vi "BBB_ParseString.vi"(8 "Input String":string) -> (1 "Spectral Data":dbl[](array[numeric]), 2 "Data out":T1, 3 "file name":string, 5 "BBB Timestamp":timestamp)   [LabVIEW 2025]
uses:
  TypeDef_DataIn.ctl
panel:
  in  "Data in":T1
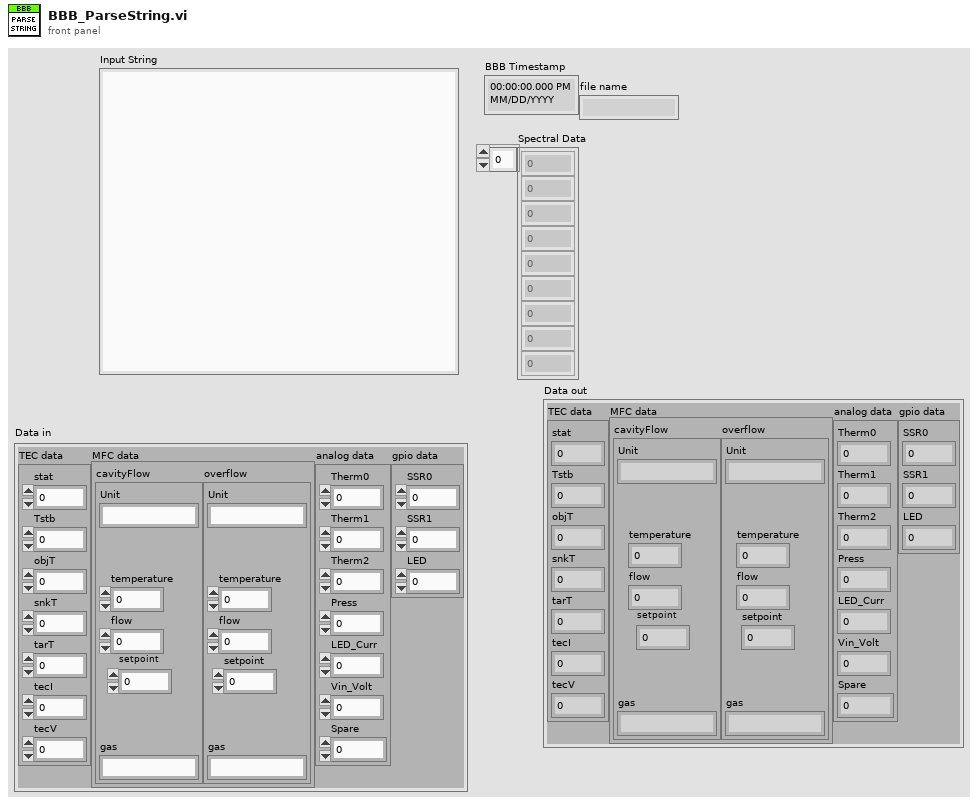
[diagram p1: front panel]
types:
  T1 = typedef "TypeDef_DataIn.ctl" = cluster{"TEC data":cluster{"stat":i32, "Tstb":i32, "objT":dbl, "snkT":dbl, "tarT":dbl, "tecI":dbl, "tecV":dbl}, "MFC data":cluster{"cavityFlow":cluster{"Unit":string, "temperature":dbl, "flow":dbl, "setpoint":dbl, "gas":string}, "overflow":cluster{"Unit":string, "temperature":dbl, "flow":dbl, "setpoint":dbl, "gas":string}}, "analog data":cluster{"Therm0":dbl, "Therm1":dbl, "Therm2":dbl, "Press":dbl, "LED_Curr":dbl, "Vin_Volt":dbl, "Spare":dbl}, "gpio data":cluster{"SSR0":i32, "SSR1":i32, "LED":i32}}
  T2 = cluster{"cavityFlow":cluster{"Unit":string, "temperature":dbl, "flow":dbl, "totalizer":dbl, "setpoint":dbl, "valve drive":dbl, "gas":string}, "overflow":cluster{"Unit":string, "temperature":dbl, "flow":dbl, "totalizer":dbl, "setpoint":dbl, "valve drive":dbl, "gas":string}}
  T3 = cluster{"stat":i32, "Tstb":i32, "objT":dbl, "snkT":dbl, "tarT":dbl, "tecI":dbl, "tecV":dbl}
  T4 = cluster{"cavityFlow":cluster{"Unit":string, "temperature":dbl, "flow":dbl, "setpoint":dbl, "gas":string}, "overflow":cluster{"Unit":string, "temperature":dbl, "flow":dbl, "setpoint":dbl, "gas":string}}
  T5 = cluster{"Therm0":dbl, "Therm1":dbl, "Therm2":dbl, "Press":dbl, "LED_Curr":dbl, "Vin_Volt":dbl, "Spare":dbl}
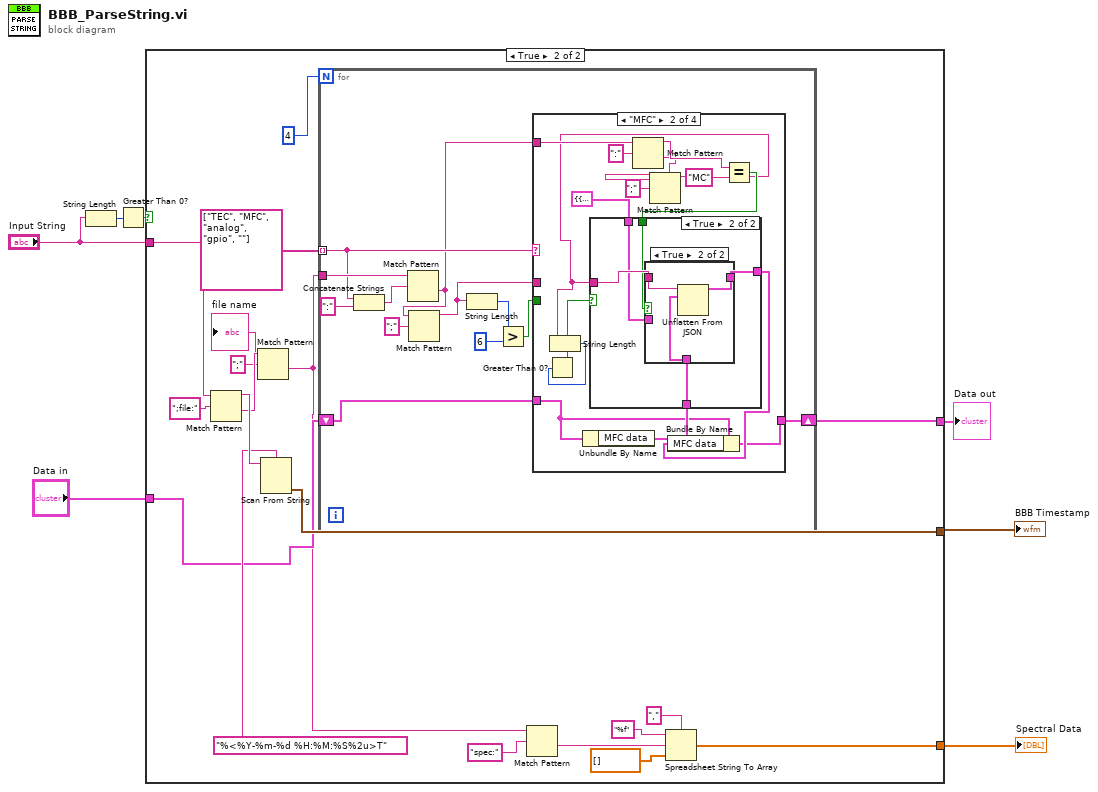
[diagram p0: block diagram]
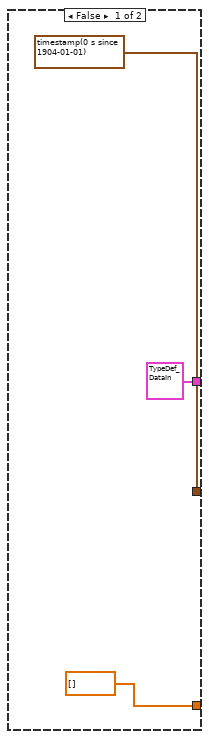
[diagram p2: hidden frame]
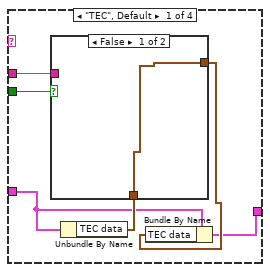
[diagram p3: hidden frame]
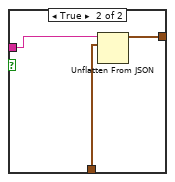
[diagram p4: hidden frame]
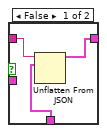
[diagram p6: hidden frame]
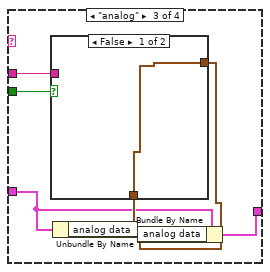
[diagram p7: hidden frame]
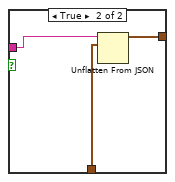
[diagram p8: hidden frame]
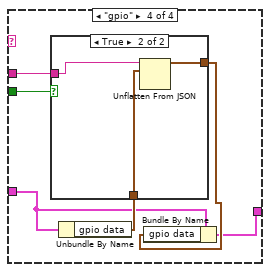
[diagram p9: hidden frame]
diagram:
  n1 = String Length(string="Input String") -> (length=w7:i32)
  n2 = Greater Than 0?(x=w7) -> (x > 0?=w6:bool)
  n3 = case shown="True" w6 {
    tunnel: "Input String" -> [_ w28]
    tunnel: [timestamp(0 s since 1904-01-01) w26] -> w4
    tunnel: [dbl[] [] ("array type (2D Dbl)") w17] -> w3
    tunnel: [T1 {"TEC data"={"stat"=0, "Tstb"=0, "objT"=0.0, "snkT"=0.0, "tarT"=0.0, "tecI"=0.0, "tecV"=0.0}, "MFC data"={"cavityFlow"={"Unit"="", "temperature"=0.0, "flow"=0.0, "setpoint"=0.0, "gas"=""}, "overflow"={"Unit"="", "temperature"=0.0, "flow"=0.0, "setpoint"=0.0, "gas"=""}}, "analog data"={"Therm0"=0.0, "Therm1"=0.0, "Therm2"=0.0, "Press"=0.0, "LED_Curr"=0.0, "Vin_Volt"=0.0, "Spare"=0.0}, "gpio data"={"SSR0"=0, "SSR1"=0, "LED"=0}} ("Data in") w16] -> w1
    tunnel: "Data in" -> [_ w15]
    frame False {
    }
    frame True {
      n4 = Match Pattern(string=w28, regular expression=";file:" ("string")) -> (before substring=w27:string, after substring=w14:string)  [unwired: 1 in, 2 out]
      n5 = Match Pattern(string=w14, regular expression=";") -> (before substring=→"file name":string, after substring=w12:string)  [unwired: 1 in, 2 out]
      n6 = Scan From String(format string="%<%Y-%m-%d %H:%M:%S%2u>T", input string=w27) -> (output 1=w26:timestamp)  [unwired: 3 in, 3 out]
      n7 = for {
        N: 4 -> [_]
        tunnel: w12 -> [w41]
        tunnel: string[] ["TEC", "MFC", "analog", "gpio", ""] -> [w36] mode=indexing
        shift-right: [w35] -> w16
        shift-left: w15 -> [w34]
        n8 = Concatenate Strings(w36, ":" ("string")) -> (w40:string)
        n9 = Match Pattern(string=w41, regular expression=w40) -> (after substring=w33:string)  [unwired: 1 in, 3 out]
        n10 = Match Pattern(string=w33, regular expression=";") -> (before substring=w37:string)  [unwired: 1 in, 3 out]
        n11 = String Length(string=w37) -> (length=w32:i32)
        n12 = Greater?(x=w32, y=6) -> (0:w30:bool)
        n13 = case shown="\"MFC\"" w36 {
          tunnel: w37 -> [w47 _ w84 w94]
          tunnel: w30 -> [w46 _ w83 w93]
          tunnel: w34 -> [w44 w65 w81 w91]
          tunnel: [w42 w63 w79 w89] -> w35
          tunnel: w33 -> [_ w58 _ _]
          frame "TEC", Default {
            n14 = Unbundle By Name(w44) -> ("TEC data"=w45:T3)
            n15 = case shown="False" w46 {
              tunnel: [w48 w51] -> w43
              tunnel: w47 -> [_ w50]
              tunnel: w45 -> [w48 w49]
              frame False {
              }
              frame True {
                n16 = Unflatten From JSON(JSON string=w50, type and defaults=w49) -> (value=w51:T3)  [unwired: 5 in, 1 out]
              }
            }
            n17 = Bundle By Name(cluster=w44, "TEC data"=w43) -> (w42:T1)
          }
          frame "MFC" {
            n18 = Unbundle By Name(w65) -> ("MFC data"=w66:T4)
            n19 = Match Pattern(string=w58, regular expression=":") -> (before substring=w57:string, after substring=w56:string)  [unwired: 1 in, 2 out]
            n20 = Match Pattern(string=w56, regular expression=";") -> (before substring=w54:string)  [unwired: 1 in, 3 out]
            n21 = String Length(string=w54) -> (length=w53:i32)
            n22 = Greater Than 0?(x=w53) -> (x > 0?=w52:bool)
            n23 = Equal?(x=w57, y="MC") -> (x = y?=w59:bool)
            n24 = case shown="True" w52 {
              tunnel: [w67 w72] -> w64
              tunnel: w54 -> [_ w71]
              tunnel: w66 -> [w67 w70]
              tunnel: T2 {"cavityFlow"={"Unit"="", "temperature"=0.0, "flow"=0.0, "totalizer"=0.0, "setpoint"=0.0, "valve drive"=0.0, "gas"=""}, "overflow"={"Unit"="", "temperature"=0.0, "flow"=0.0, "totalizer"=0.0, "setpoint"=0.0, "valve drive"=0.0, "gas"=""}} ("MFC data") -> [_ w69]
              tunnel: w59 -> [_ w68]
              frame False {
              }
              frame True {
                n25 = case shown="True" w68 {
                  tunnel: [w75 w78] -> w72
                  tunnel: w71 -> [w74 w77]
                  tunnel: w70 -> [w73 w76]
                  tunnel: w69 -> [_ _]
                  frame False {
                    n26 = Unflatten From JSON(JSON string=w74, type and defaults=w73) -> (value=w75:T4)  [unwired: 5 in, 1 out]
                  }
                  frame True {
                    n27 = Unflatten From JSON(JSON string=w77, type and defaults=w76) -> (value=w78:T4)  [unwired: 5 in, 1 out]
                  }
                }
              }
            }
            n28 = Bundle By Name(cluster=w65, "MFC data"=w64) -> (w63:T1)
          }
          frame "analog" {
            n29 = Unbundle By Name(w81) -> ("analog data"=w82:T5)
            n30 = case shown="False" w83 {
              tunnel: [w85 w88] -> w80
              tunnel: w84 -> [_ w87]
              tunnel: w82 -> [w85 w86]
              frame False {
              }
              frame True {
                n31 = Unflatten From JSON(JSON string=w87, type and defaults=w86) -> (value=w88:T5)  [unwired: 5 in, 1 out]
              }
            }
            n32 = Bundle By Name(cluster=w81, "analog data"=w80) -> (w79:T1)
          }
          frame "gpio" {
            n33 = Unbundle By Name(w91) -> ("gpio data"=w92:cluster{"SSR0":i32, "SSR1":i32, "LED":i32})
            n34 = case shown="True" w93 {
              tunnel: [w95 w98] -> w90
              tunnel: w94 -> [_ w97]
              tunnel: w92 -> [w95 w96]
              frame False {
              }
              frame True {
                n35 = Unflatten From JSON(JSON string=w97, type and defaults=w96) -> (value=w98:cluster{"SSR0":i32, "SSR1":i32, "LED":i32})  [unwired: 5 in, 1 out]
              }
            }
            n36 = Bundle By Name(cluster=w91, "gpio data"=w90) -> (w89:T1)
          }
        }
      }
      n37 = Match Pattern(string=w12, regular expression="spec:") -> (after substring=w18:string)  [unwired: 1 in, 3 out]
      n38 = Spreadsheet String To Array(delimiter (Tab)=",", format string="%f", spreadsheet string=w18, array type (2D Dbl)=dbl[] []) -> (array=w17:dbl[])
    }
  }
  "Spectral Data" <- w3
  "BBB Timestamp" <- w4
  "Data out" <- w1
